vi "Model - DeInit.vi"(8 "error in (no error)":errorcluster, 11 "View Model":T1) -> (0 "error out":errorcluster)   [LabVIEW 2017]
doc: "De-Initialize central data/events storage of MVC."
uses:
  Controls/View Model.ctl
  Controls/Shared Model.ctl
  Error Handler/Controls/Error Model.ctl
  Error Handler/Controls/Error Message.ctl
  Error Handler/Controls/Error Level.ctl
  Configuration/Controls/Database Model.ctl
  Configuration/Controls/Database Message.ctl
  Configuration/Controls/Database Command.ctl
  Configuration/Controls/Database Overhead.ctl
  Configuration/Controls/Database Status.ctl
  Configuration/Controls/Database Record.ctl
  Configuration/Controls/Database - Rule Record.ctl
  Controller/Controls/CNTRLR - Wash Step.ctl
  Controller/Controls/CNTRLR - Position.ctl
  Controller/Controls/CNTRLR - Model.ctl
  Controller/Controls/CNTRLR - Message.ctl
  Controller/Controls/CNTRLR - Command.ctl
  Controller/Controls/CNTRLR - Overhead.ctl
  Controller/Controls/CNTRLR - State.ctl
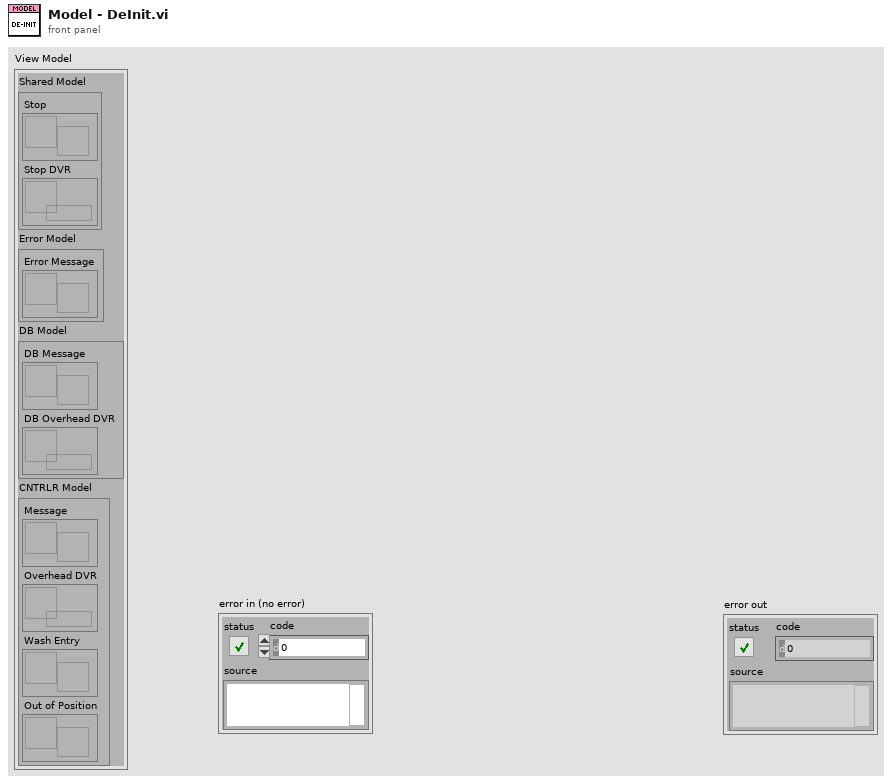
[diagram p1: front panel]
types:
  T1 = typedef "View Model.ctl" = cluster{"Shared Model":T2, "Error Model":T3, "DB Model":T4, "CNTRLR Model":T5}
  T2 = typedef "Shared Model.ctl" = cluster{"Stop":refnum<user-event>, "Stop DVR":refnum<data-value>}
  T3 = typedef "Error Model.ctl" = cluster{"Error Message":refnum<user-event>}
  T4 = typedef "Database Model.ctl" = cluster{"DB Message":refnum<user-event>, "DB Overhead DVR":refnum<data-value>}
  T5 = typedef "CNTRLR - Model.ctl" = cluster{"Message":refnum<user-event>, "Overhead DVR":refnum<data-value>, "Wash Entry":refnum<user-event>, "Out of Position":refnum<user-event>}
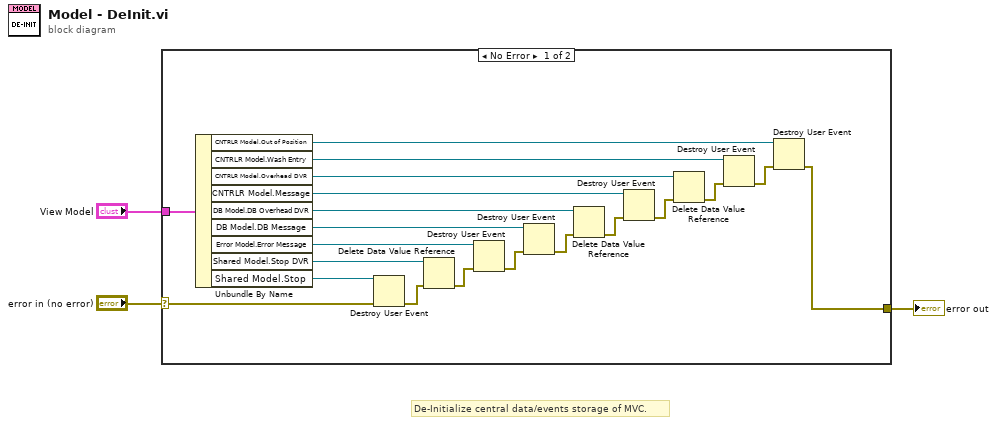
[diagram p0: block diagram]
diagram:
  # "De-Initialize central data/events storage of MVC."
  n1 = case shown="No Error" "error in (no error)" {
    selector: "error in (no error)" -> [w5 w24]
    tunnel: [w4 w24] -> w2
    tunnel: "View Model" -> [w23 _]
    frame No Error {
      n2 = Unbundle By Name(w23) -> ("CNTRLR Model.Out of Position"=w7:refnum<user-event>, "CNTRLR Model.Wash Entry"=w9:refnum<user-event>, "CNTRLR Model.Overhead DVR"=w11:refnum<data-value>, "CNTRLR Model.Message"=w13:refnum<user-event>, "DB Model.DB Overhead DVR"=w15:refnum<data-value>, "DB Model.DB Message"=w17:refnum<user-event>, "Error Model.Error Message"=w19:refnum<user-event>, "Shared Model.Stop DVR"=w21:refnum<data-value>, "Shared Model.Stop"=w22:refnum<user-event>)
      n3 = Destroy User Event(user event=w22, error in=w5) -> (error out=w20:errorcluster)
      n4 = Delete Data Value Reference(data value reference=w21, error in=w20) -> (error out=w18:errorcluster)  [unwired: 1 out]
      n5 = Destroy User Event(user event=w19, error in=w18) -> (error out=w16:errorcluster)
      n6 = Destroy User Event(user event=w17, error in=w16) -> (error out=w14:errorcluster)
      n7 = Delete Data Value Reference(data value reference=w15, error in=w14) -> (error out=w12:errorcluster)  [unwired: 1 out]
      n8 = Destroy User Event(user event=w13, error in=w12) -> (error out=w10:errorcluster)
      n9 = Delete Data Value Reference(data value reference=w11, error in=w10) -> (error out=w8:errorcluster)  [unwired: 1 out]
      n10 = Destroy User Event(user event=w9, error in=w8) -> (error out=w6:errorcluster)
      n11 = Destroy User Event(user event=w7, error in=w6) -> (error out=w4:errorcluster)
    }
    frame Error {
    }
  }
  "error out" <- w2
